vi "Do.vi"(8 "error in (no error)":errorcluster, 10 "DataExchange":T1, 11 "DataLogger in":refnum<class "DataLogger.lvclass">) -> (0 "error out":errorcluster, 2 "DataExchange Out":T1, 3 "DataLogger out":refnum<class "DataLogger.lvclass">)   [LabVIEW 2020, in "DataLogger.lvlib" / "DataLogger.lvclass"]
uses:
  DataLogger.lvclass
  Hardware Abstraction Layer/Component/Device/Device/DataExchange.ctl
  <vilib>/vision/Image Controls.llb/IMAQ Image.ctl
  DataProcessor/DataProcessor/DataProcessor.lvclass
  Interface/DataListener/DataListener.lvclass
panel:
  out "Source":string
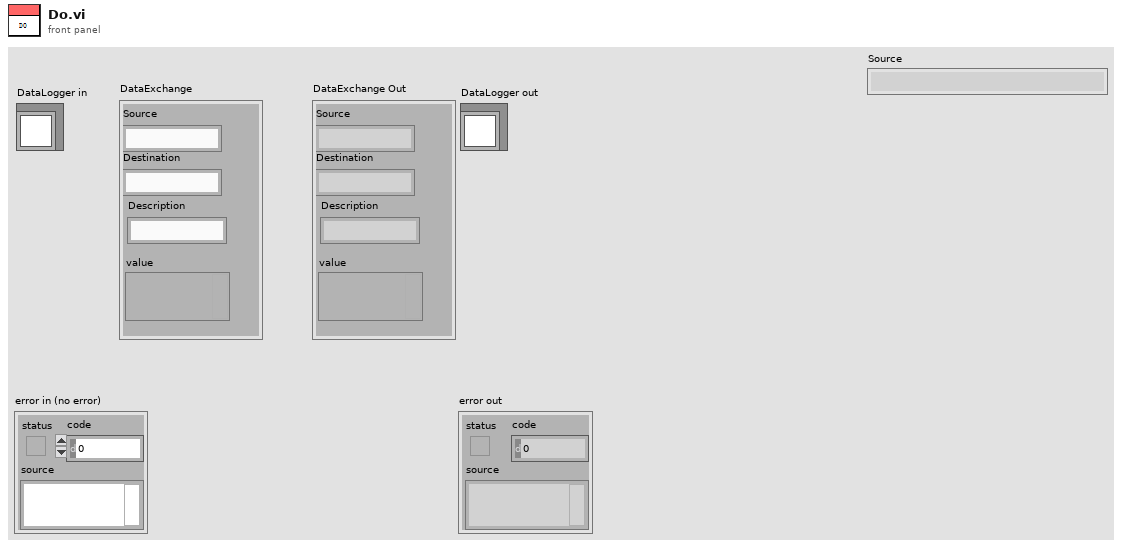
[diagram p1: front panel]
types:
  T1 = typedef "DataListener.lvclass/DataExchange.ctl" = cluster{"Source":string, "Destination":string, "Description":string, "value":variant}
  T2 = typedef "IMAQ Image.ctl" = refnum<image>
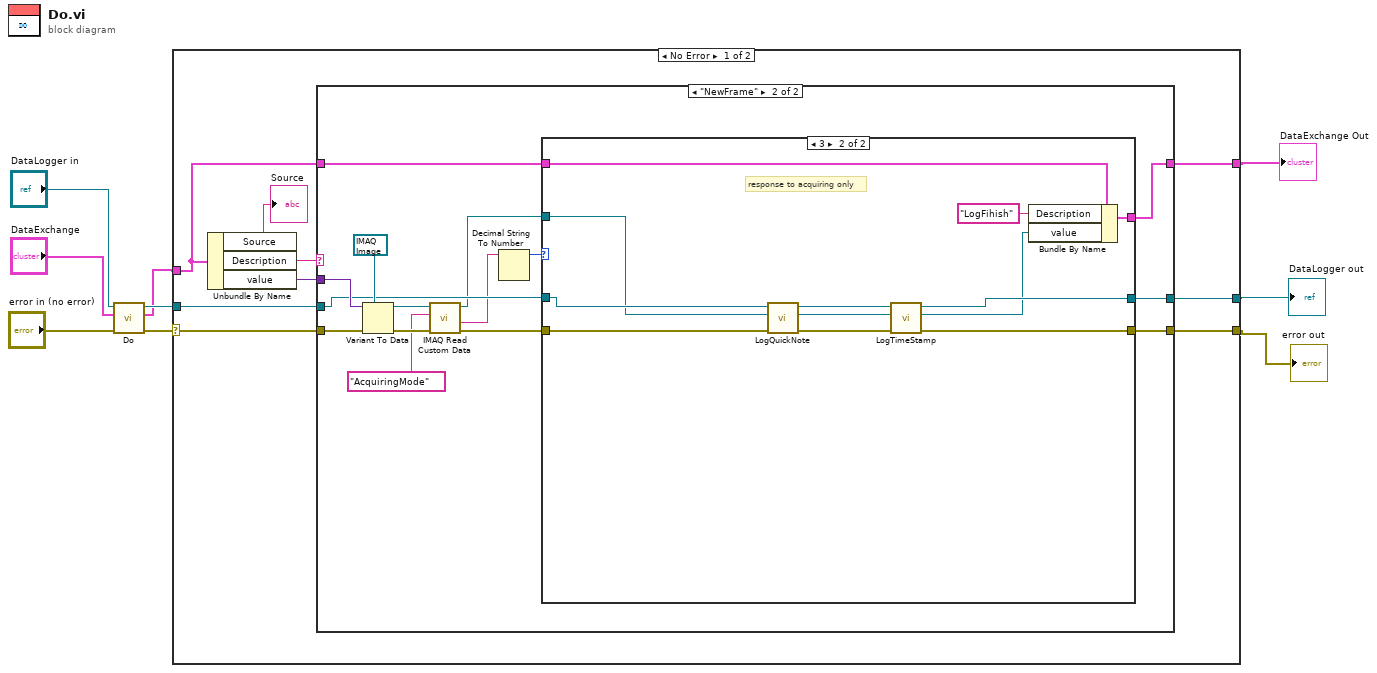
[diagram p0: block diagram]
diagram:
  n1 = call-parent "Do.vi"("error in (no error)"="error in (no error)", "DataExchange"="DataExchange", "DataProcessor in"="DataLogger in") -> ("error out"=w6:errorcluster, "DataExchange Out"=w4:T1, "DataProcessor out"=w5:refnum<class "DataLogger.lvclass">)  [unwired: 6 in]
  n2 = case shown="No Error" w6 {
    selector: w6 -> [w16 w54]
    tunnel: [w17 w54] -> w3
    tunnel: w5 -> [w13 w53]
    tunnel: [w18 w53] -> w2
    tunnel: w4 -> [w12 w52]
    tunnel: [w11 w52] -> w1
    frame No Error {
      n3 = Unbundle By Name(w12) -> ("Source"=→"Source":string, "Description"=w15:string, "value"=w14:variant)
      n4 = case shown="\"NewFrame\"" w15 {
        tunnel: w14 -> [_ w35]
        tunnel: [w21 w25] -> w18
        tunnel: w13 -> [w21 w26]
        tunnel: [w20 w27] -> w17
        tunnel: w16 -> [w20 w36]
        tunnel: w12 -> [w19 w32]
        tunnel: [w19 w31] -> w11
        frame Default {
        }
        frame "NewFrame" {
          n5 = Variant To Data(error in=w36, type=T2 refnum ("New Image"), Variant=w35) -> (data=w29:T2, error out=w33:errorcluster)
          n6 = call "IMAQ Read Custom Data"("error in (no error)"=w33, "Key"="AcquiringMode", "Image"=w29) -> ("error out"=w30:errorcluster, "Custom Data Out"=w23:string, "Image (duplicate)"=w24:T2)  [unwired: 6 in]
          n7 = Decimal String To Number(string=w23) -> (number=w22:i32)  [unwired: 2 in, 1 out]
          n8 = case shown="3" w22 {
            tunnel: w32 -> [w39 w51]
            tunnel: [w39 w50] -> w31
            tunnel: w30 -> [w37 w49]
            tunnel: w24 -> [_ w46]
            tunnel: [w37 w44] -> w27
            tunnel: w26 -> [w38 w47]
            tunnel: [w38 w42] -> w25
            frame Default {
            }
            frame 3 {
              # "response to acquiring only"
              n9 = call-dynamic "LogQuickNote.vi"("error in (no error)"=w49, "New Image"=w46, "DataLogger in"=w47) -> ("error out"=w48:errorcluster, "Image Out"=w41:T2, "DataLogger out"=w43:refnum<class "DataLogger.lvclass">)  [unwired: 6 in]
              n10 = call-dynamic "LogTimeStamp.vi"("error in (no error)"=w48, "New Image"=w41, "DataLogger in"=w43) -> ("error out"=w44:errorcluster, "Image Out"=w40:T2, "DataLogger out"=w42:refnum<class "DataLogger.lvclass">)  [unwired: 6 in]
              n11 = Bundle By Name(cluster=w51, "Description"="LogFihish", "value"=w40) -> (w50:T1)
            }
          }
        }
      }
    }
    frame Error {
    }
  }
  "error out" <- w3
  "DataLogger out" <- w2
  "DataExchange Out" <- w1
